vi "PARTs_CameraBackground Loop.vi"(11 "CameraDevRef":T1) -> ()   [LabVIEW 2015]
doc: "This VI acquires the image buffer from the camera MJPG stream at the configured fps rate. It notifies any waiting VIs and allows them to pick up the latest image. This allows the camera and robot vision loop to run at different rates. The 1011, camera is far more efficient using MJPGs, and generally, this is probably the better choice for the camera loop.\n \nThis software is licensed. Open the labview\\readme\\WPI Robotics Library Open Source License.txt file for more information."
uses:
  <vilib>/Rock Robotics/WPI/Camera/WPI_CameraDevRef.ctl
  <vilib>/Rock Robotics/WPI/Camera/WPI_CameraSettings Operations.ctl
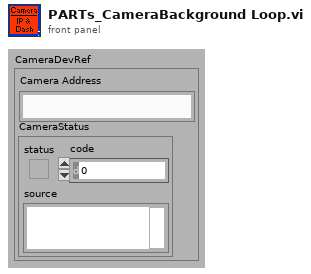
[diagram p1: front panel]
types:
  T1 = typedef "WPI_CameraDevRef.ctl" = cluster{"Camera Address":string, "CameraStatus":errorcluster}
  T2 = typedef "WPI_CameraSettings Operations.ctl" = enum16{"Udate FPS", "Update Compression", "Update Size", "Update White Balance", "Update Brightness", "Update Sharpness", "Update Exposure", "Update Exposure Value", "Update Color Level", "Update Exp Priority", "Update Color Enable", "Update JPG", "Update MJPG", "Read and Clear", "Read", "Init"}
  T3 = typedef "WPI_CameraSettings Control.ctl" = cluster{"FPS":i32, "Compression":i32, "Size":i32, "White Balance":i32, "Brightness":i32, "Sharpness":i32, "Exposure":i32, "Color Level":i32, "Exposure Priority":i32, "Color Enable":i32, "JPG Loop":i32, "MJPG Loop":i32, "Exposure Value":i32}
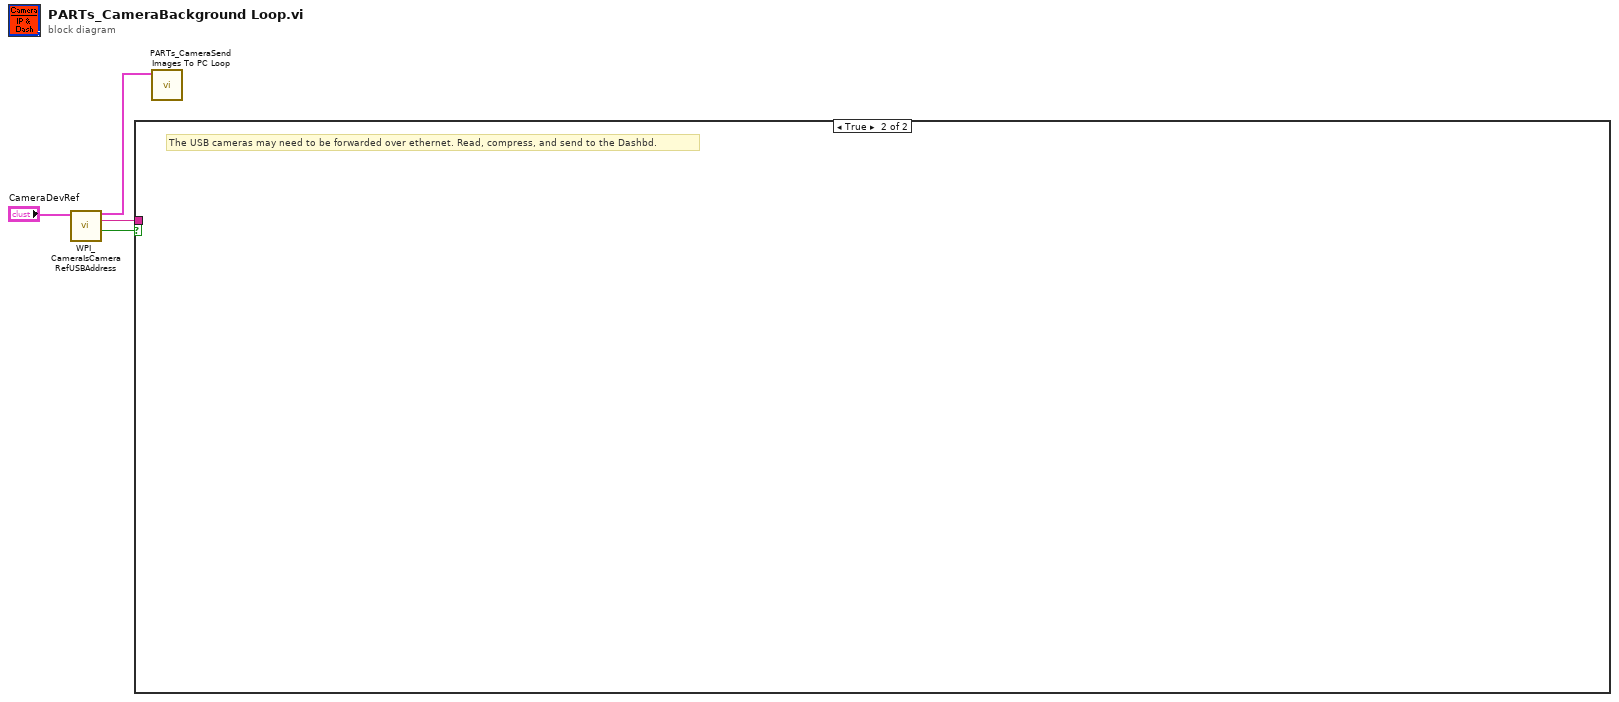
[diagram p0: block diagram]
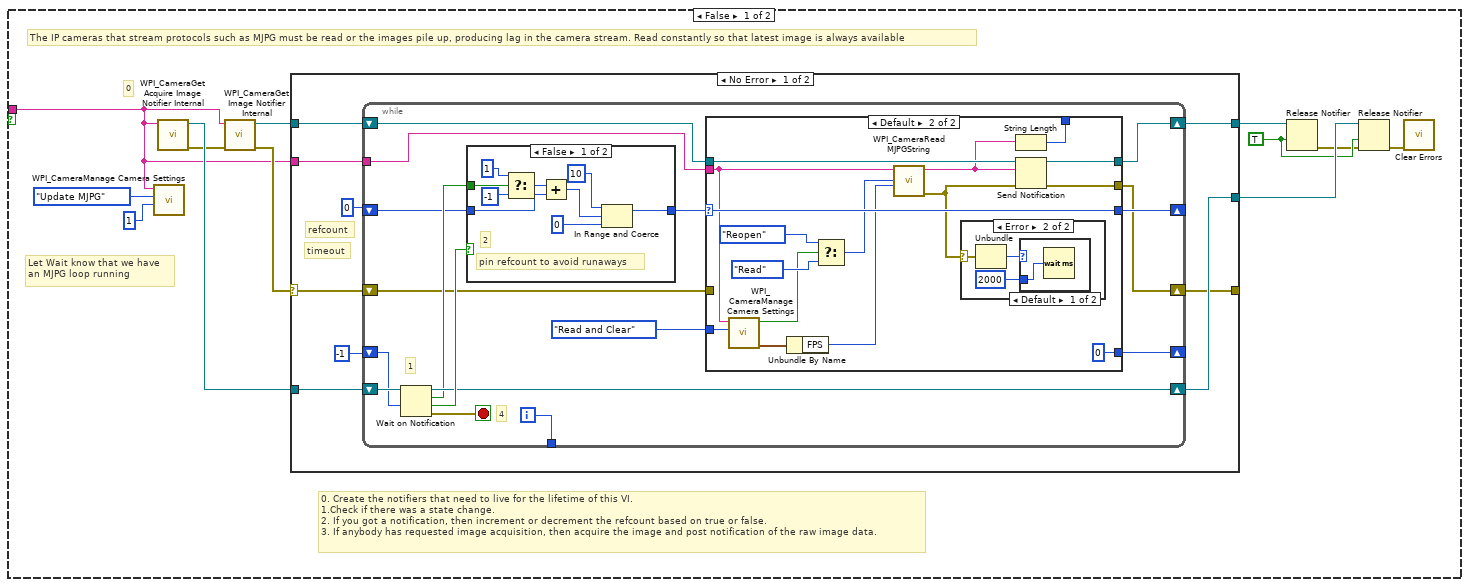
[diagram p2: hidden frame]
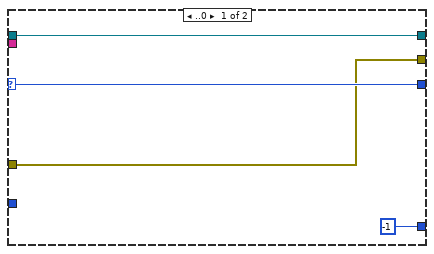
[diagram p3: hidden frame]
diagram:
  n1 = call <vilib>:"WPI_CameraIsCameraRefUSBAddress.vi"("CameraDevRef"="CameraDevRef") -> ("USB?"=w3:bool, "Camera Address Out"=w2:string, "CameraDevRef out"=w1:T1)  [unwired: 7 in, 1 out]
  n2 = case shown="True" w3 {
    tunnel: w2 -> [w6 _]
    frame False {
      w13 = TRUE ("force destroy? (F)")
      # "The IP cameras that stream protocols such as MJPG must be read or the images pile up, producing lag in the camera stream. Read constantly so that latest image is always available"
      # "0. Create the notifiers that need to live for the lifetime of this VI. \n1.Check if there was a state change.\n2. If you got a notification, then increment or decrement the refcount based on true or false.\n3. If anybody has requested image acquisition, then acquire the image and post notification of the raw image data."
      # "Let Wait know that we have\nan MJPG loop running"
      # "0"
      n3 = call <vilib>:"WPI_CameraManage Camera Settings.vi"("Value"=1, "Operation"=WPI_CameraSettings_Operations."Update MJPG", "Camera IP"=w6) -> ()  [unwired: 7 in, 2 out]
      n4 = call <vilib>:"WPI_CameraGet Acquire Image Notifier Internal.vi"("Camera Address"=w6) -> ("error out"=w10:errorcluster, "Acquire Image Notifier"=w11:refnum<notifier>)  [unwired: 1 in, 8 out]
      n5 = call <vilib>:"WPI_CameraGet Image Notifier Internal.vi"("error in (no error)"=w10, "Camera Address"=w6) -> ("error out"=w12:errorcluster, "Image Notifier"=w14:refnum<notifier>)  [unwired: 8 out]
      n6 = case shown="No Error" w12 {
        selector: w12 -> [w18 w79]
        tunnel: w6 -> [w25 _]
        tunnel: w11 -> [w24 w77]
        tunnel: w14 -> [w22 w78]
        tunnel: [w20 w78] -> w16
        tunnel: [w19 w77] -> w15
        tunnel: [w17 w79] -> _
        frame No Error {
          # "timeout"
          # "refcount"
          n7 = while {
            shift-right: [w40] -> w19
            shift-left: w24 -> [w42]
            tunnel: w25 -> [w37]
            shift-right: [w29] -> _
            shift-left: 0 -> [w38]
            shift-right: [w35] -> w20
            shift-left: w22 -> [w36]
            shift-right: [w33] -> _
            shift-left: -1 -> [w34]
            shift-right: [w28] -> w17
            shift-left: w18 -> [w31]
            tunnel: [w26] -> _
            i -> [w26]
            stop <- w32 stop-if-true
            # "4"
            # "1"
            n8 = Wait on Notification(notifier=w42, timeout in ms (-1)=w34) -> (notifier out=w40:refnum<notifier>, notification=w39:bool, timed out?=w41:bool, error out=w32:errorcluster)  [unwired: 1 in, 1 out]
            n9 = case shown="False" w41 {
              tunnel: w39 -> [w75 _]
              tunnel: w38 -> [w71 w76]
              tunnel: [w67 w76] -> w30
              frame False {
                # "pin refcount to avoid runaways"
                # "2"
                n10 = Select(t=1, s=w75, f=-1) -> (s? t:f=w72:i32)
                n11 = Add(x=w72, y=w71) -> (x+y=w68:i32)
                n12 = In Range and Coerce(upper limit=10, x=w68, lower limit=0) -> (coerced(x)=w67:i32)  [unwired: 1 out]
              }
              frame True {
              }
            }
            n13 = case shown="Default" w30 {
              selector: w30 -> [w45 w59]
              tunnel: w37 -> [_ w47]
              tunnel: w36 -> [w46 w62]
              tunnel: [w46 w61] -> w35
              tunnel: [-1 0] -> w33
              tunnel: w31 -> [w43 _]
              tunnel: [w45 w59] -> w29
              tunnel: [w43 w58] -> w28
              tunnel: [_ w52] -> _
              tunnel: WPI_CameraSettings_Operations."Read and Clear" ("Operation") -> [_ w48]
              frame ..0 {
              }
              frame Default {
                n14 = call <vilib>:"WPI_CameraManage Camera Settings.vi"("Operation"=w48, "Camera IP"=w47) -> ("Values"=w50:T3, "Changed"=w51:bool)  [unwired: 8 in]
                n15 = Unbundle By Name(w50) -> ("FPS"=w49:i32)
                n16 = Select(t=enum16{"Read", "Reopen", "Close"}."Reopen" ("Operation"), s=w51, f=enum16{"Read", "Reopen", "Close"}."Read" ("Operation")) -> (s? t:f=w54:enum16{"Read", "Reopen", "Close"})
                n17 = call <vilib>:"WPI_CameraRead MJPGString.vi"("fps"=w49, "Operation"=w54, "address"=w47) -> ("error out"=w57:errorcluster, "Raw Image Data"=w53:string)  [unwired: 7 in]
                n18 = case shown="Error" w57 {
                  selector: w57 -> [_ w65]
                  frame No Error {
                  }
                  frame Error {
                    n19 = Unbundle(w65) -> ("code"=w64:i32)  [unwired: 2 out]
                    n20 = case shown="Default" w64 {
                      tunnel: u32 2000 ("milliseconds to wait") -> [w66 _]
                      frame Default {
                        n21 = Wait (ms)(milliseconds to wait=w66) -> ()  [unwired: 1 out]
                      }
                      frame 56 {
                      }
                    }
                  }
                }
                n22 = String Length(string=w53) -> (length=w52:i32)
                n23 = Send Notification(notification=w53, notifier=w62, error in (no error)=w57) -> (notifier out=w61:refnum<notifier>, error out=w58:errorcluster)
              }
            }
          }
        }
        frame Error {
        }
      }
      n24 = Release Notifier(notifier=w16, force destroy? (F)=w13) -> (error out=w9:errorcluster)  [unwired: 1 in, 2 out]
      n25 = Release Notifier(notifier=w15, force destroy? (F)=w13, error in (no error)=w9) -> (error out=w5:errorcluster)  [unwired: 2 out]
      n26 = call <vilib>:"Clear Errors.vi"("error in (no error)"=w5) -> ()  [unwired: 1 in, 6 out]
    }
    frame True {
      # "The USB cameras may need to be forwarded over ethernet. Read, compress, and send to the Dashbd."
    }
  }
  n27 = call "PARTs_CameraSend Images To PC Loop.vi"("CameraDevRef"=w1) -> ()  [unwired: 11 in]
